vi "Read csv teraterm configs.vi"(8 "error in (no error)":errorcluster, 9 "Use this console":u32=1 min=1 step=1, 10 "Use this config":string, 11 "Path":path=path "L:/teraterm/console_configs.csv") -> (0 "error out":errorcluster, 1 "Consoles":i32, 2 "Config database":string[][](array[string]), 3 "Config name":string, 4 "Options":T1)   [LabVIEW 2013]
uses:
  Test Support VI/Tera term Serial options.ctl
  <vilib>/Utility/file.llb/Read From Spreadsheet File (string).vi
panel:
  in  "Config Names":u16(ring) items=["Select Config", "1002213", "1234567"]
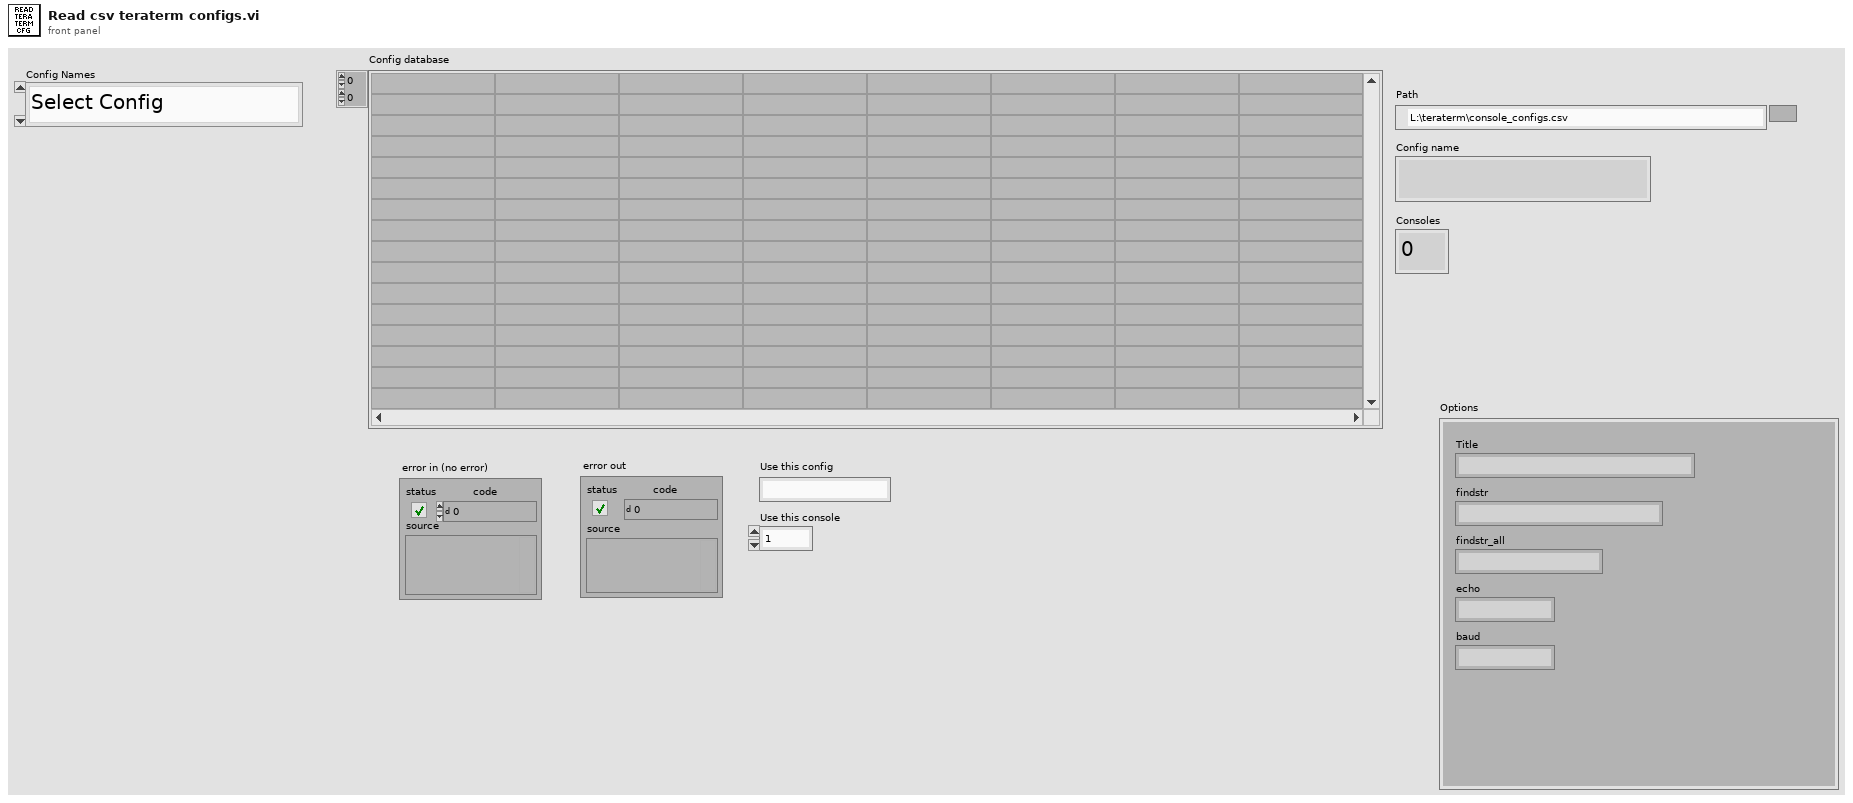
[diagram p1: front panel]
types:
  T1 = typedef "Tera term Serial options.ctl" = cluster{"Title":string, "findstr":string, "findstr_all":string, "echo":string, "baud":string}
  T2 = cluster{"Title":string, "findstr":string, "findstr_all":string, "echo":string, "baud":string}
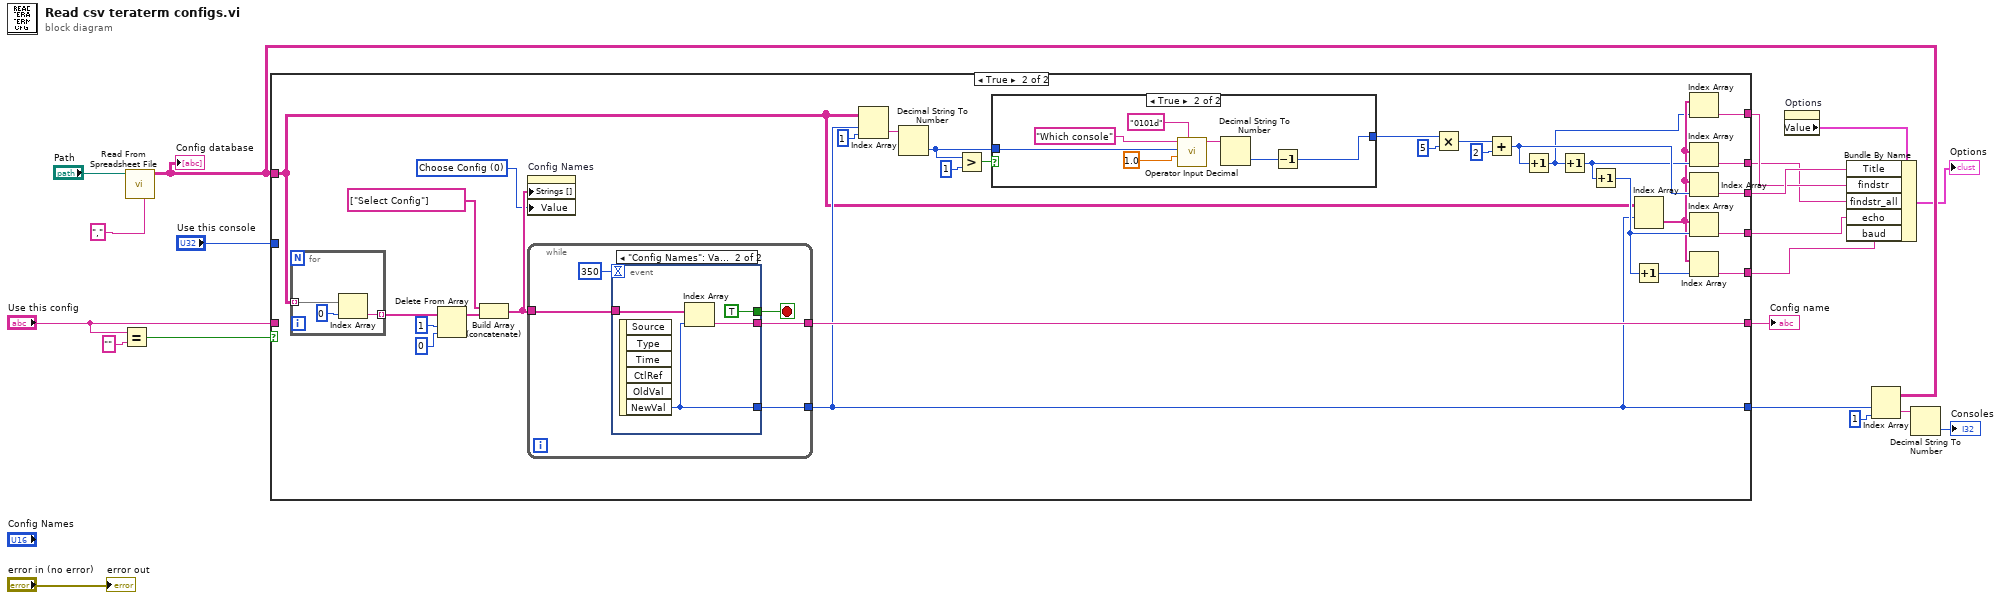
[diagram p0: block diagram]
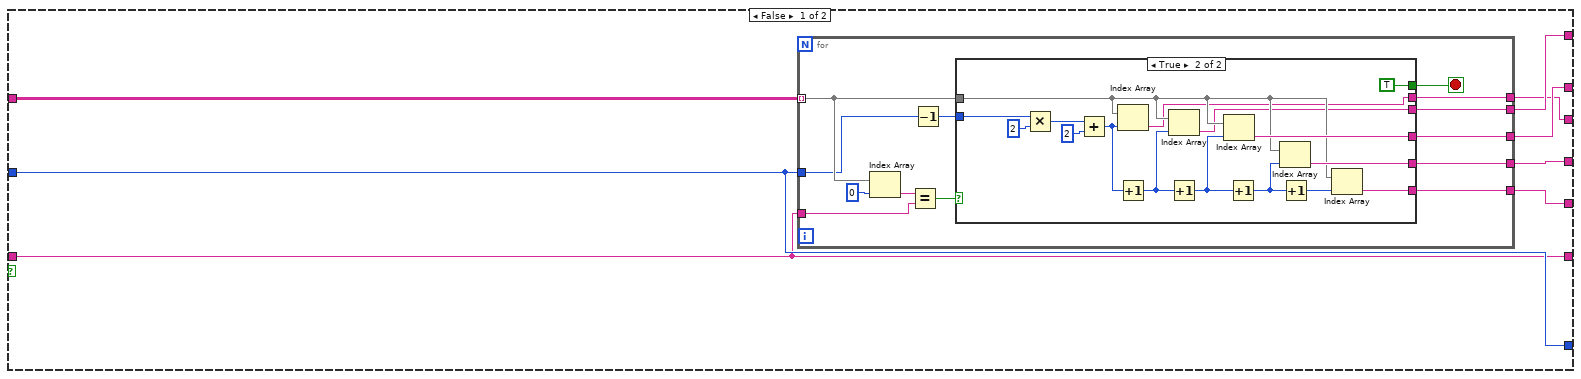
[diagram p2: hidden frame]
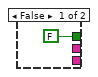
[diagram p3: hidden frame]
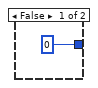
[diagram p4: hidden frame]
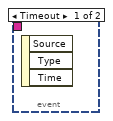
[diagram p5: hidden frame]
diagram:
  n1 = Equal?(x="Use this config", y="") -> (x = y?=w10:bool)
  n2 = call-poly <vilib>:"Read From Spreadsheet File.vi"("delimiter (\\t)"="," ("delimiter (\\t)"), "file path (dialog if empty)"="Path") -> ("all rows"=w17:string[][])  [unwired: 5 in, 4 out]
  "Config database" <- w17
  n3 = case shown="True" w10 {
    tunnel: [w26 w83] -> w19
    tunnel: w17 -> [w28 w63]
    tunnel: [w27 w70] -> w12
    tunnel: "Use this config" -> [w26 _]
    tunnel: "Use this console" -> [w27 _]
    tunnel: [w25 w60] -> w5
    tunnel: [w24 w73] -> w3
    tunnel: [w23 w72] -> w2
    tunnel: [w22 w74] -> w4
    tunnel: [w21 w64] -> w6
    frame False {
      n4 = for {
        tunnel: w28 -> [w38] mode=indexing
        tunnel: w26 -> [w34]
        tunnel: w27 -> [w37]
        tunnel: [w33] -> w25
        tunnel: [w32] -> w24
        tunnel: [w31] -> w23
        tunnel: [w30] -> w22
        tunnel: [w29] -> w21
        stop <- w35 stop-if-true
        n5 = Index Array(array=w38, index=0) -> (element=w40:string)
        n6 = Equal?(x=w40, y=w34) -> (x = y?=w39:bool)
        n7 = Decrement(x=w37) -> (x-1=w36:u32)
        n8 = case shown="True" w39 {
          tunnel: w38 -> [_ w47]
          tunnel: w36 -> [_ w58]
          tunnel: [FALSE TRUE] -> w35
          tunnel: [_ w43] -> w33
          tunnel: [_ w50] -> w32
          tunnel: [_ w49] -> w31
          tunnel: [_ w48] -> w30
          tunnel: [_ w46] -> w29
          frame False {
          }
          frame True {
            n9 = Multiply(x=w58, y=u32 2) -> (x*y=w56:u32)
            n10 = Add(x=w56, y=u32 2) -> (x+y=w54:u32)
            n11 = Index Array(array=w47, index=w54) -> (element=w46:string)
            n12 = Increment(x=w54) -> (x+1=w45:u32)
            n13 = Index Array(array=w47, index=w45) -> (element=w43:string)
            n14 = Increment(x=w45) -> (x+1=w44:u32)
            n15 = Index Array(array=w47, index=w44) -> (element=w48:string)
            n16 = Increment(x=w44) -> (x+1=w53:u32)
            n17 = Index Array(array=w47, index=w53) -> (element=w50:string)
            n18 = Increment(x=w53) -> (x+1=w52:u32)
            n19 = Index Array(array=w47, index=w52) -> (element=w49:string)
          }
        }
      }
    }
    frame True {
      w81 = u16 0 items=["Choose Config", "1002213", "1234567"] ("Config Names")
      n20 = for {
        tunnel: w63 -> [w108] mode=indexing
        tunnel: [w106] -> w88 mode=indexing
        n21 = Index Array(array=w108, index=0) -> (element=w106:string)
      }
      n22 = Delete From Array(array=w88, length=1, index=0) -> (array with subset deleted=w84:string[])  [unwired: 1 out]
      n23 = Build Array (concatenate)(string[] ["Select Config"] ("element"), w84) -> (w82:string[])
      n24 = property on="Config Names" class="Ring (strict)"("Strings []"=w82, "Value"=w81) -> ()  [unwired: 2 in, 2 out]
      n25 = while {
        tunnel: w82 -> [w101]
        tunnel: [w100] -> w83
        tunnel: [w97] -> w70
        stop <- w99 stop-if-true
        n26 = event shown="[1] \"Config Names\": Value Change" {
          selector: _ -> [_ _]
          dyn-events: _ -> [_ _]
          timeout: 350 -> [_ _]
          tunnel: w101 -> [_ w103]
          tunnel: [_ w105] -> w100
          tunnel: [_ TRUE] -> w99
          tunnel: [_ w102] -> w97
          event Timeout {
            n27 = event-data() -> ()  [unwired: 1 in, 3 out]
          }
          event "Config Names": Value Change {
            n28 = event-data() -> ("NewVal"=w102:u16)  [unwired: 1 in, 5 out]
            n29 = Index Array(array=w103, index=w102) -> (element=w105:string)
          }
        }
      }
      n30 = Index Array(array=w63, index (row)=w70, index (col)=1 ("disabled index (col)")) -> (element=w68:string)
      n31 = Decimal String To Number(string=w68) -> (number=w66:i32)  [unwired: 2 in, 1 out]
      n32 = Greater?(x=w66, y=1) -> (0:w67:bool)
      n33 = case shown="True" w67 {
        tunnel: w66 -> [_ w96]
        tunnel: [0 w91] -> w65
        frame False {
        }
        frame True {
          n34 = call "Operator Input Decimal.vi"("Data format"="0101d", "Lower limit"=1.0, "Upper limit"=w96, "Message"="Which console") -> ("Response"=w94:string)  [unwired: 4 in, 3 out]
          n35 = Decimal String To Number(string=w94) -> (number=w92:i32)  [unwired: 2 in, 1 out]
          n36 = Decrement(x=w92) -> (x-1=w91:i32)
        }
      }
      n37 = Multiply(x=w65, y=u32 5) -> (x*y=w79:u32)
      n38 = Add(x=w79, y=u32 2) -> (x+y=w77:u32)
      n39 = Increment(x=w77) -> (x+1=w59:u32)
      n40 = Increment(x=w59) -> (x+1=w62:u32)
      n41 = Increment(x=w62) -> (x+1=w76:u32)
      n42 = Increment(x=w76) -> (x+1=w75:u32)
      n43 = Index Array(array=w63, index (row)=w70) -> (element=w61:string[])  [unwired: 1 in]
      n44 = Index Array(array=w61, index=w59) -> (element=w60:string)
      n45 = Index Array(array=w61, index=w62) -> (element=w74:string)
      n46 = Index Array(array=w61, index=w77) -> (element=w64:string)
      n47 = Index Array(array=w61, index=w76) -> (element=w73:string)
      n48 = Index Array(array=w61, index=w75) -> (element=w72:string)
    }
  }
  "Config name" <- w19
  n49 = property on="Options" class="Clust (strict)"() -> ("Value"=w7:T2)  [unwired: 2 in, 2 out]
  n50 = Bundle By Name(cluster=w7, "Title"=w6, "findstr"=w5, "findstr_all"=w4, "echo"=w3, "baud"=w2) -> (→"Options":T2)
  n51 = Index Array(array=w17, index (row)=w12, index (col)=1 ("disabled index (col)")) -> (element=w15:string)
  n52 = Decimal String To Number(string=w15) -> (number=→"Consoles":i32)  [unwired: 2 in, 1 out]
  "error out" <- "error in (no error)"
